vi "WD_AS_add_new.vi"(8 "error in (no error)":errorcluster, 10 "New data":cluster{"條碼A":string, "條碼B":string}, 11 "DBLink":string="Driver={ODBC Driver 17 for SQL Server};Server=localhost\\SQLEXPRESS;Database=ZDX201;UID=labview;PWD=Dsa@54137926") -> (0 "error out":errorcluster, 1 "站點總數":i32, 2 "當前料數":i32, 3 "計算用 array":cluster{"條碼A":string, "條碼B":string}[](array[cluster]), 5 "顯示用array":cluster{"條碼A":string, "條碼B":string}[](array[cluster]))   [LabVIEW 2019]
panel:
  out "x-y":i32
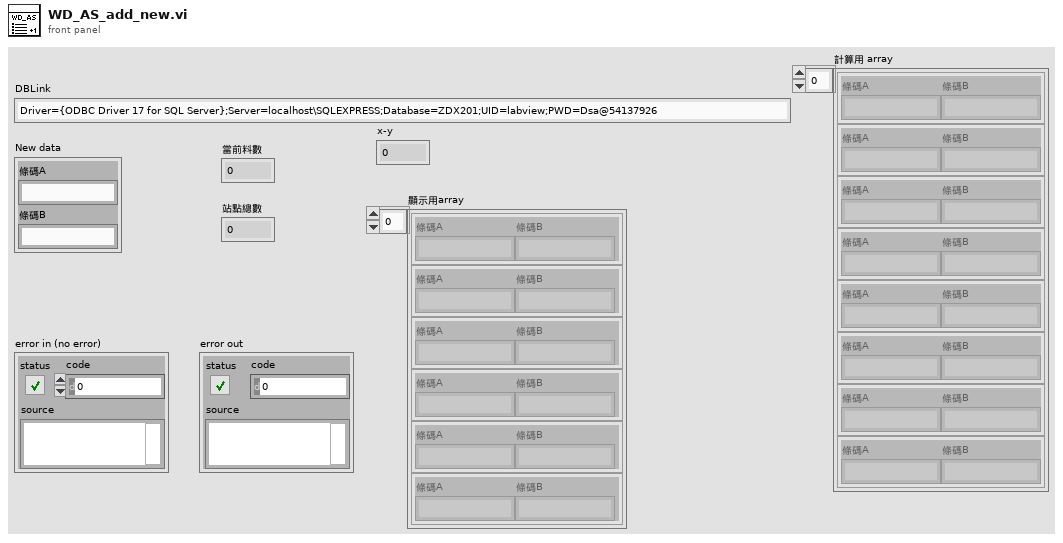
[diagram p1: front panel]
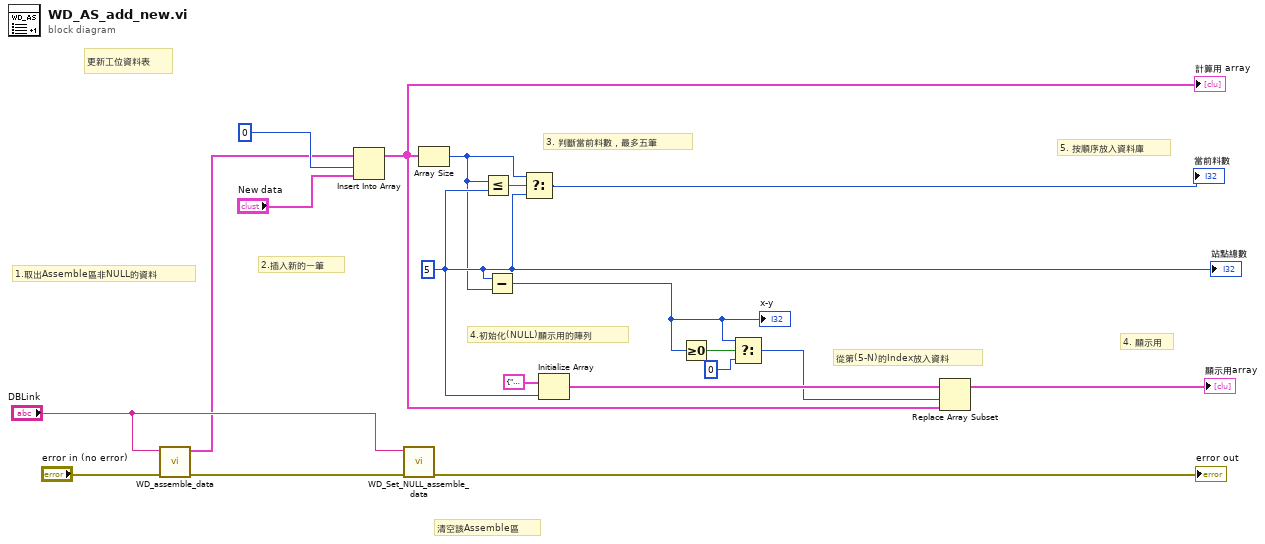
[diagram p0: block diagram]
diagram:
  w9 = 5
  # "從第(5-N)的Index放入資料"
  # "4.初始化(NULL)顯示用的陣列"
  # "3. 判斷當前料數，最多五筆"
  # "5. 按順序放入資料庫"
  # "4. 顯示用"
  # "清空該Assemble區"
  # "2.插入新的一筆"
  # "1.取出Assemble區非NULL的資料"
  # "更新工位資料表"
  n1 = call "WD_assemble_data.vi"("error in (no error)"="error in (no error)", "DBlink"="DBLink") -> ("error out"=w15:errorcluster, "Workplace: assemble"=w1:cluster{"條碼A":string, "條碼B":string}[])  [unwired: 6 in, 2 out]
  n2 = Insert Into Array(array=w1, index=0, new element="New data") -> (w10:cluster{"條碼A":string, "條碼B":string}[])
  "計算用 array" <- w10
  n3 = call "WD_Set_NULL_assemble_data.vi"("error in (no error)"=w15, "DBlink"="DBLink") -> ("error out"=→"error out":errorcluster)  [unwired: 8 in, 1 out]
  n4 = Array Size(array=w10) -> (size(s)=w8:i32)
  n5 = Less Or Equal?(x=w8, y=w9) -> (x <= y?=w18:bool)
  n6 = Subtract(x=w9, y=w8) -> (x-y=w3:i32)
  "x-y" <- w3
  n7 = Select(t=w8, s=w18, f=w9) -> (s? t:f=→"當前料數":i32)
  n8 = Initialize Array(cluster{"條碼A":string, "條碼B":string} {"條碼A"="NULL", "條碼B"="NULL"} ("New data"), w9) -> (w11:cluster{"條碼A":string, "條碼B":string}[])
  n9 = Greater Or Equal To 0?(x=w3) -> (x >= 0?=w5:bool)
  n10 = Select(t=w3, s=w5, f=i16 0) -> (s? t:f=w2:i32)
  n11 = Replace Array Subset(array=w11, new element=w10, index=w2) -> (→"顯示用array":cluster{"條碼A":string, "條碼B":string}[])
  "站點總數" <- w9
